vi "Write ReportEvent.vi"(10 "Report Event":refnum<user-event>, 11 "Test Report.Default in":refnum<class "Test Report.Event.lvclass">) -> (3 "Test Report.Default out":refnum<class "Test Report.Event.lvclass">)   [LabVIEW 2013, in "Caraya.lvlib" / "Test Report.Event.lvclass"]
uses:
  Test Report.Event.lvclass
  Test Report.Event.lvclass/Test Report.Event.ctl
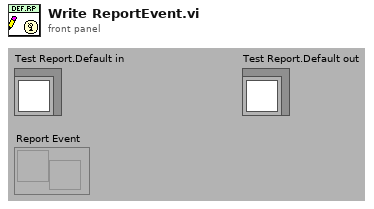
[diagram p1: front panel]
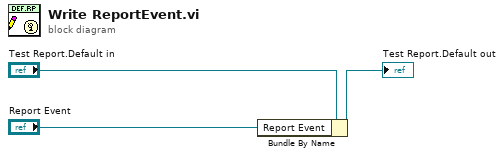
[diagram p0: block diagram]
diagram:
  n1 = Bundle By Name(cluster="Test Report.Default in", "Report Event"="Report Event") -> (→"Test Report.Default out":refnum<class "Test Report.Event.lvclass">)
